vi "1-Rotina de aquisição dos dados de caracterização.vi"() -> ()   [LabVIEW 2011]
uses:
  <vilib>/Instr/_visa.llb/VISA Configure Serial Port (Instr).vi
panel:
  in  "Delay (ms)":u32
  out "submatrix":dbl[][](array[numeric])
  out "Gráfico 2":dbl[](graph)
  out "Delay real (ms)":u32
  out "Tempo decorrido(s)":dbl caption="Elapsed Time (s)"
  in  "Parar programa":bool
  in  "OK Button":bool
  out "direito":dbl
  out "esquerdo":dbl
  out "Gráfico2":dbl[](graph)
  in  "Parar Aquisição do Sinal":bool
  out "String Concatenada":string
  in  "baud rate":u32=9600
  in  "VISA resource name":refnum<visa-resource-name>
  # "ROTINA DE AQUISI敲O DOS DADOS DE CARACTERIZA敲O"
  # "SINAL AQUISITADO EM TEMPO REAL"
  # "VISA Resourse Name:"
  # "Baud Rate:"
  # "Delay:"
  # "ms"
  # "ms"
  # "Delay sofrido em cada iteração:"
  # "Tempo de Aquisição Decorrido:"
  # "s"
  # "SINAL A SER GRAVADO PARA PROCESSAMENTO"
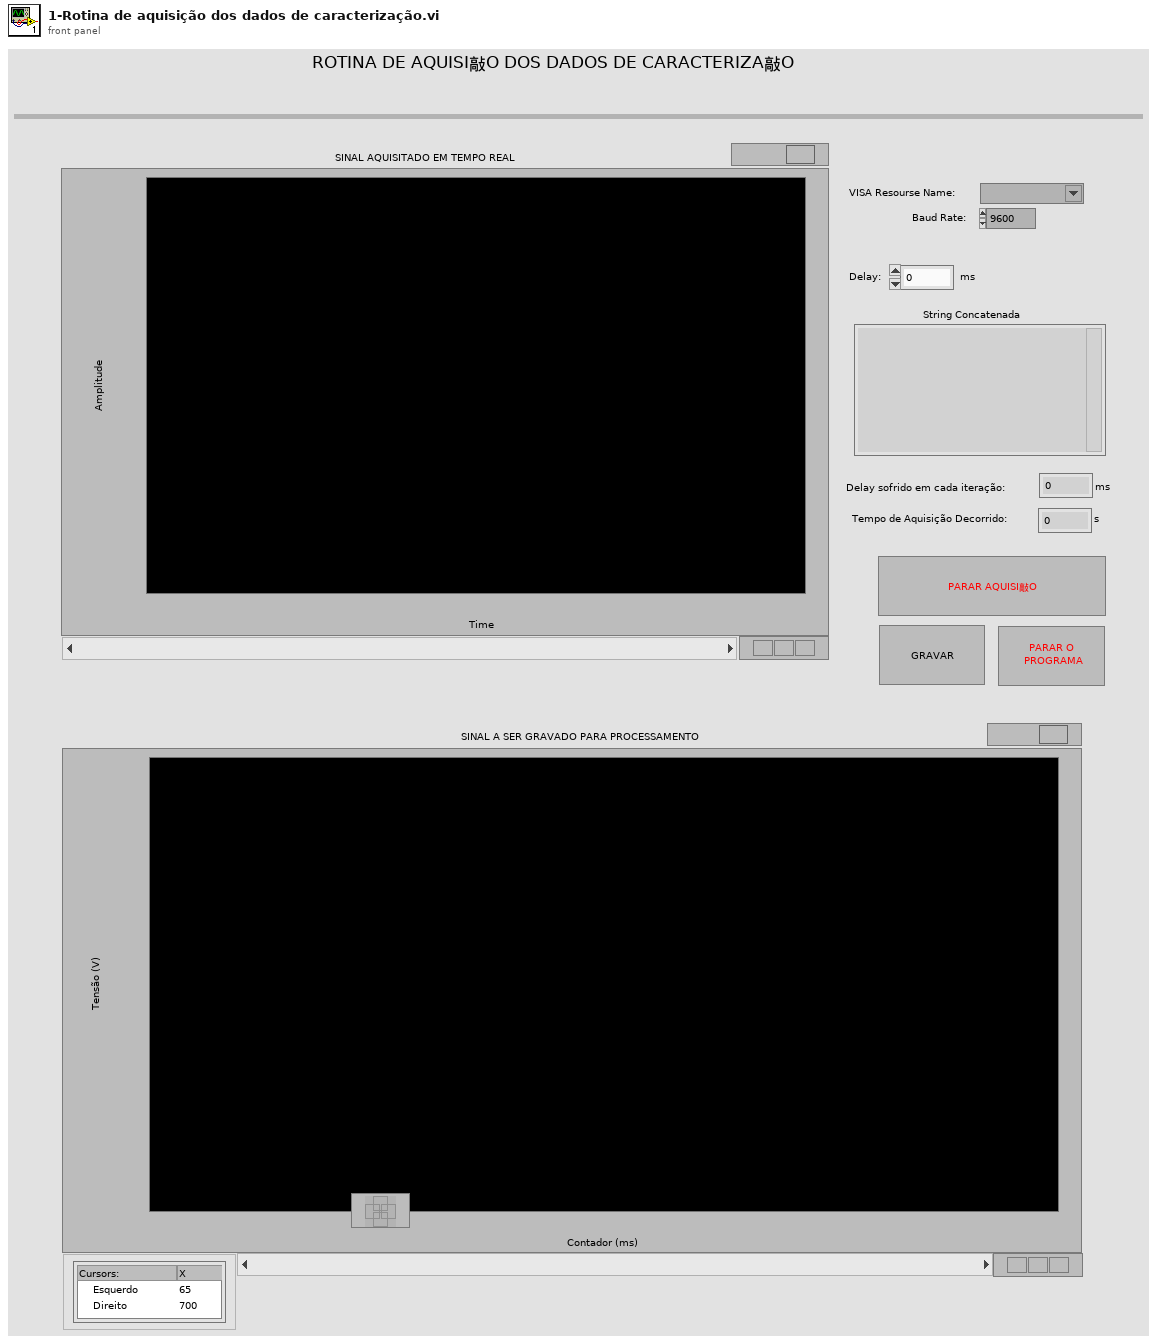
[diagram p1: front panel]
types:
  T1 = typedef "NI_Matrix.lvlib/RealMatrix.ctl" = dbl[][]
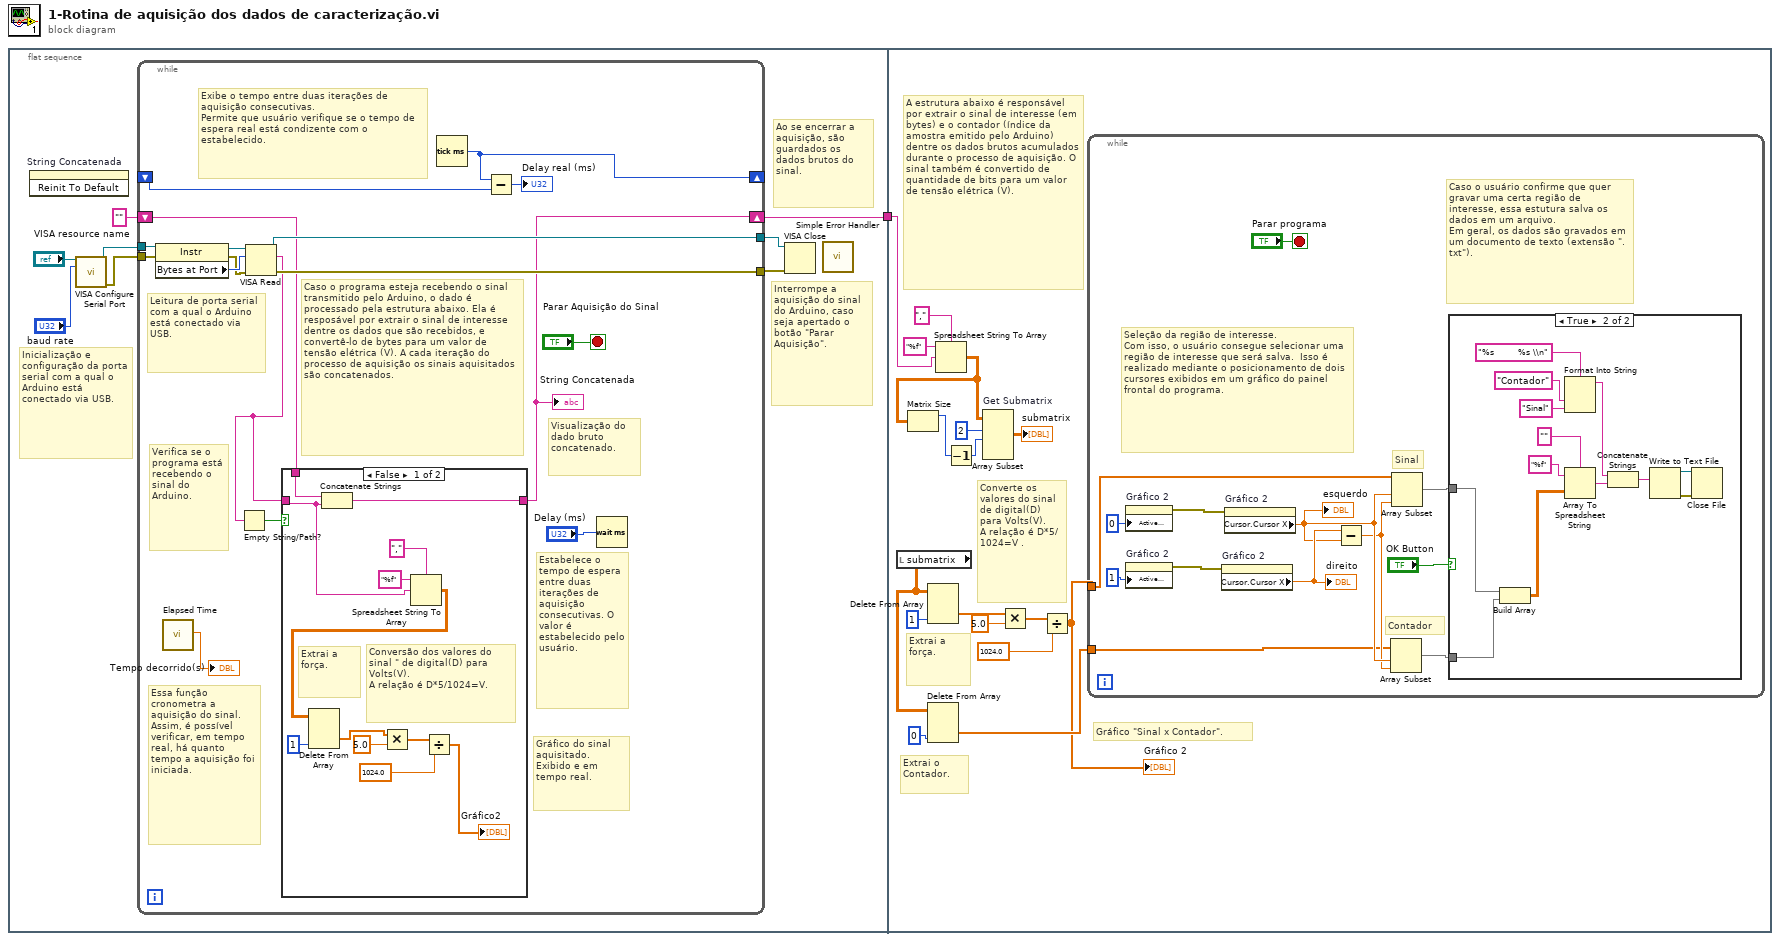
[diagram p0: block diagram]
diagram:
  n1 = flat-sequence {
    tunnel: [w4] -> w1
    tunnel: w1 -> [w43]
    frame #0 {
      # "Interrompe a aquisição do sinal do Arduino, caso seja apertado o botão \"Parar Aquisição\"."
      # "Ao se encerrar a aquisição, são guardados os dados brutos do sinal."
      # "Inicialização e configuração da porta serial com a qual o Arduino está conectado via USB."
      n2 = invoke on="String Concatenada" class="Str" method="Reinit To Default"() -> ()  [unwired: 3 in, 3 out]
      n3 = call-poly "VISA Configure Serial Port"("VISA resource name"="VISA resource name", "baud rate (9600)"="baud rate") -> ("VISA resource name out"=w9:refnum<visa-resource-name>, "error out"=w8:errorcluster)  [unwired: 12 in]
      n4 = while {
        tunnel: w9 -> [w26]
        tunnel: w8 -> [w25]
        tunnel: [w22] -> w3
        tunnel: [w21] -> w2
        shift-right: [w12] -> w4
        shift-left: "" -> [w14]
        shift-right: [w17] -> _
        shift-left: _ -> [w18]
        stop <- "Parar Aquisição do Sinal" stop-if-true
        # "Visualização do dado bruto concatenado."
        # "Caso o programa esteja recebendo o sinal transmitido pelo Arduino, o dado é processado pela estrutura abaixo. Ela é resposável por extrair o sinal de interesse dentre os dados que são recebidos, e convertê-lo de bytes para um valor de tensão elétrica (V). A cada iteração do processo de aquisição os sinais aquisitados são concatenados."
        # "Exibe o tempo entre duas iterações de aquisição consecutivas. \nPermite que usuário verifique se o tempo de espera real está condizente com o estabelecido."
        # "Gráfico do sinal aquisitado. Exibido e em tempo real."
        # "Leitura de porta serial com a qual o Arduino está conectado via USB."
        # "Verifica se o programa está recebendo o sinal do Arduino."
        # "Essa função cronometra a aquisição do sinal. Assim, é possível verificar, em tempo real, há quanto tempo a aquisição foi iniciada."
        # "Estabelece o tempo de espera entre duas iterações de aquisição consecutivas. O valor é estabelecido pelo usuário."
        n5 = property class="Instr"(reference=w26, error in=w25) -> (reference out=w24:refnum<visa-resource-name>, error out=w19:errorcluster, "Bytes at Port"=w23:u32)
        n6 = call "Elapsed Time"() -> ("Elapsed Time (s)"=→"Tempo decorrido(s)":dbl)  [unwired: 12 in, 7 out]
        n7 = VISA Read(VISA resource name=w24, byte count=w23, error in (no error)=w19) -> (VISA resource name out=w22:refnum<visa-resource-name>, read buffer=w13:string, error out=w21:errorcluster)  [unwired: 1 out]
        n8 = Empty String/Path?(string/path=w13) -> (empty?=w15:bool)
        n9 = case shown="False" w15 {
          tunnel: w14 -> [w38 w39]
          tunnel: w13 -> [w33 _]
          tunnel: [w37 w39] -> w12
          frame False {
            # "Conversão dos valores do sinal \" de digital(D) para Volts(V).\nA relação é D*5/1024=V."
            # "Extrai a força."
            n10 = Concatenate Strings(w38, w33) -> (w37:string)
            n11 = Spreadsheet String To Array(delimiter (Tab)=",", format string="%f", spreadsheet string=w33) -> (array=w34:dbl[][])  [unwired: 1 in]
            n12 = Delete From Array(array=w34, index (col)=1 ("disabled index (col)")) -> (deleted portion=w29:dbl[])  [unwired: 2 in, 1 out]
            n13 = Multiply(x=w29, y=5.0) -> (x*y=w31:dbl[])
            n14 = Divide(x=w31, y=1024.0) -> (x/y=→"Gráfico2":dbl[])
          }
          frame True {
          }
        }
        "String Concatenada" <- w12
        n15 = Tick Count (ms)() -> (millisecond timer value=w17:u32)
        n16 = Subtract(x=w17, y=w18) -> (x-y=→"Delay real (ms)":u32)
        n17 = Wait (ms)(milliseconds to wait="Delay (ms)") -> ()  [unwired: 1 out]
      }
      n18 = VISA Close(VISA resource name=w3, error in (no error)=w2) -> ()  [unwired: 1 out]
      n19 = call <vilib>:"Simple Error Handler.vi"() -> ()  [unwired: 2 in, 8 out]
    }
    frame #1 {
      # "Gráfico \"Sinal x Contador\"."
      # "Converte os valores do sinal de digital(D) para Volts(V).\nA relação é D*5/1024=V ."
      # "A estrutura abaixo é responsável por extrair o sinal de interesse (em bytes) e o contador (índice da amostra emitido pelo Arduino) dentre os dados brutos acumulados durante o processo de aquisição. O sinal também é convertido de quantidade de bits para um valor de tensão elétrica (V)."
      # "Extrai o Contador."
      # "Extrai a força."
      n20 = local read "submatrix"() -> (w48:dbl[][])
      n21 = Delete From Array(array=w48, index (col)=1 ("disabled index (col)")) -> (deleted portion=w44:dbl[])  [unwired: 2 in, 1 out]
      n22 = Delete From Array(array=w48, index (col)=0 ("disabled index (col)")) -> (deleted portion=w42:dbl[])  [unwired: 2 in, 1 out]
      n23 = Spreadsheet String To Array(delimiter (Tab)=",", format string="%f", spreadsheet string=w43) -> (array=w54:dbl[][])  [unwired: 1 in]
      n24 = Matrix Size(0:w54) -> (1:w52:i32)  [unwired: 1 out]
      n25 = Decrement(x=w52) -> (x-1=w51:i32)
      n26 = Array Subset "Get Submatrix"(array=w54, index (row)=2, length (row)=w51) -> (→"submatrix":dbl[][])  [unwired: 2 in]
      n27 = Multiply(x=w44, y=5.0) -> (x*y=w46:dbl[])
      n28 = Divide(x=w46, y=1024.0) -> (x/y=w41:dbl[])
      "Gráfico 2" <- w41
      n29 = while {
        tunnel: w42 -> [w59]
        tunnel: w41 -> [w57]
        stop <- "Parar programa" stop-if-true
        # "Caso o usuário confirme que quer gravar uma certa região de interesse, essa estutura salva os dados em um arquivo.\nEm geral, os dados são gravados em um documento de texto (extensão \".txt\")."
        # "Seleção da região de interesse. \nCom isso, o usuário consegue selecionar uma região de interesse que será salva.  Isso é realizado mediante o posicionamento de dois cursores exibidos em um gráfico do painel frontal do programa."
        # "Contador"
        # "Sinal"
        n30 = property on="Gráfico 2" class="WFGraph (strict)"("Active Cursor"=u32 0) -> (error out=w69:errorcluster)  [unwired: 2 in, 1 out]
        n31 = property on="Gráfico 2" class="WFGraph (strict)"("Active Cursor"=u32 1) -> (error out=w67:errorcluster)  [unwired: 2 in, 1 out]
        n32 = property on="Gráfico 2" class="WFGraph (strict)"(error in=w67) -> ("Cursor.Cursor X"=w65:dbl)  [unwired: 1 in, 2 out]
        "direito" <- w65
        n33 = property on="Gráfico 2" class="WFGraph (strict)"(error in=w69) -> ("Cursor.Cursor X"=w61:dbl)  [unwired: 1 in, 2 out]
        "esquerdo" <- w61
        n34 = Subtract(x=w65, y=w61) -> (x-y=w60:dbl)
        n35 = Array Subset(array=w59, index=w61, length=w60) -> (w58:dbl[])
        n36 = Array Subset(array=w57, index=w61, length=w60) -> (w63:dbl[])
        n37 = case shown="True" "OK Button" {
          tunnel: w63 -> [_ w82]
          tunnel: w58 -> [_ w81]
          frame False {
          }
          frame True {
            n38 = Build Array(w82, w81) -> (w70:T1)
            n39 = Format Into String(format string="%s        %s \\n", "Contador" ("input 1"), "Sinal" ("input 2")) -> (resulting string=w77:string)  [unwired: 2 in, 1 out]
            n40 = Array To Spreadsheet String(delimiter (Tab)="", array=w70, 3:"%f" ("format string")) -> (spreadsheet string=w76:string)
            n41 = Concatenate Strings(w77, w76) -> (w80:string)
            n42 = Write to Text File(text=w80) -> (refnum out=w78:refnum<file>, error out=w79:errorcluster)  [unwired: 3 in, 1 out]
            n43 = Close File(refnum=w78, error in=w79) -> ()  [unwired: 2 out]
          }
        }
      }
    }
  }
